vi "Create Pattern Script(OM).vi"(8 "error in (no error)":errorcluster, 10 "BML OM":T1, 11 "BML Pattern Creater in":refnum<class "BML Pattern Creater.lvclass">) -> (0 "error out":errorcluster, 2 "OM string out":string, 3 "BML Pattern Creater out":refnum<class "BML Pattern Creater.lvclass">)   [LabVIEW 2018, in "BML Pattern Creater.lvlib" / "BML Pattern Creater.lvclass"]
uses:
  BML Pattern Creater.lvclass
  Ctls/OM - BML.ctl
  Interfaces/Protocol Interface.lvlibp/Interfaces/Protocol Interface/Pin State.ctl
  Interfaces/Protocol Interface.lvlibp/Interfaces/Protocol Interface/Protocol Interface.lvclass
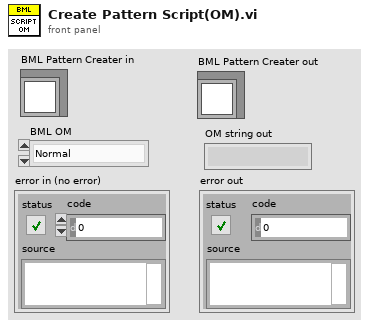
[diagram p1: front panel]
types:
  T1 = typedef "OM - BML.ctl" = enum16{"Normal", "ImmeEffect", "InitSlaveID", "LoadData"}
  T2 = typedef "Protocol Interface.lvlibp/Protocol Interface.lvclass/Pin State.ctl" = enum16{"0", "1", "L", "H", "X", "V", "D", "M"}
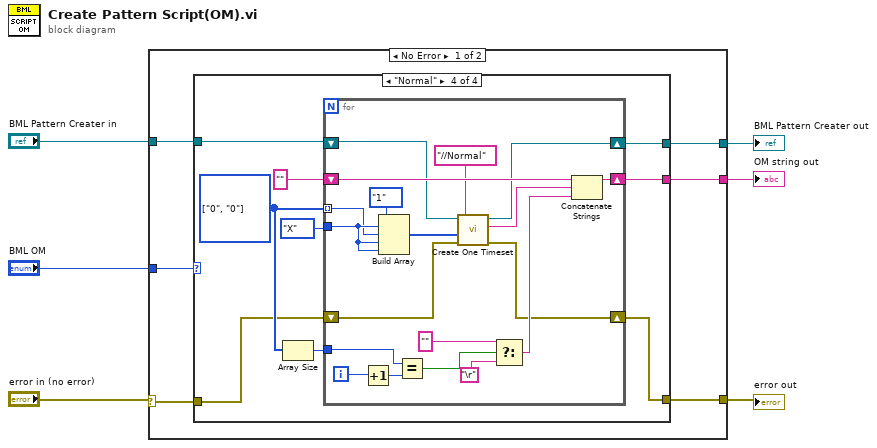
[diagram p0: block diagram]
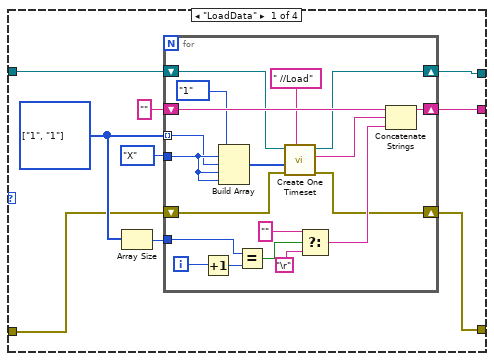
[diagram p2: hidden frame]
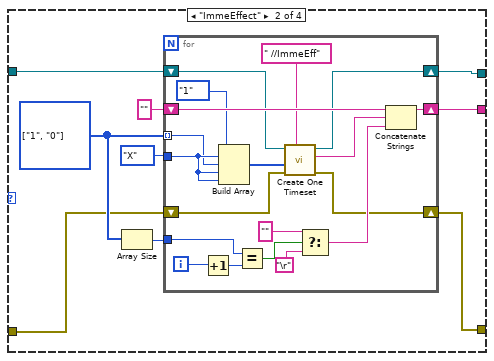
[diagram p3: hidden frame]
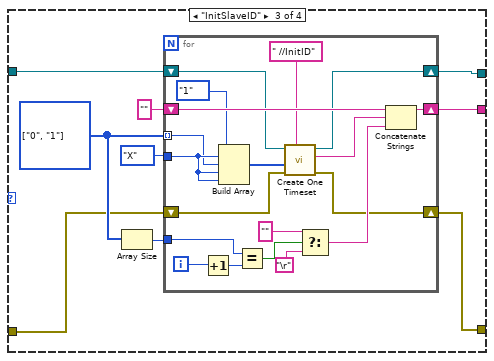
[diagram p4: hidden frame]
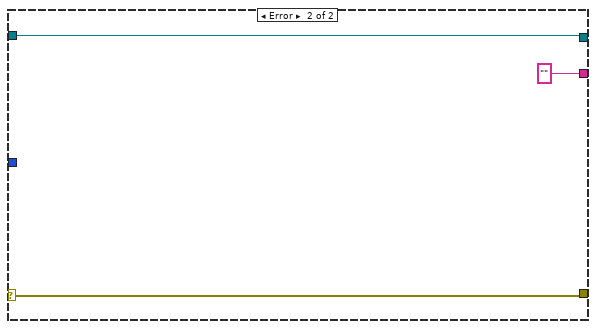
[diagram p5: hidden frame]
diagram:
  n1 = case shown="No Error" "error in (no error)" {
    selector: "error in (no error)" -> [w10 w126]
    tunnel: "BML OM" -> [w12 _]
    tunnel: [w11 "" ("string out")] -> w5
    tunnel: [w9 w126] -> w4
    tunnel: "BML Pattern Creater in" -> [w8 w125]
    tunnel: [w7 w125] -> w1
    frame No Error {
      n2 = case shown="\"Normal\"" w12 {
        tunnel: [w20 w48 w76 w104] -> w11
        tunnel: w10 -> [w16 w44 w72 w100]
        tunnel: [w14 w42 w70 w99] -> w9
        tunnel: w8 -> [w15 w43 w71 w97]
        tunnel: [w13 w41 w69 w98] -> w7
        frame "LoadData" {
          w19 = T2[] [enum."1", enum."1"] items=["0", "1", "L", "H", "X", "V", "D", "M"] ("PinState")
          n3 = Array Size(array=w19) -> (size(s)=w18:i32)
          n4 = for {
            tunnel: w19 -> [w30] mode=indexing
            shift-right: [w39] -> w20
            shift-left: "" ("string out") -> [w40]
            tunnel: w18 -> [w37]
            tunnel: Pin_State."X" ("PinState") -> [w31]
            shift-right: [w24] -> w14
            shift-left: w16 -> [w25]
            shift-right: [w22] -> w13
            shift-left: w15 -> [w23]
            i -> [w38]
            n5 = Increment(x=w38) -> (x+1=w36:i32)
            n6 = Build Array(Pin_State."1" ("PinState"), w31, w30, w31, w31) -> (w26:T2[])
            n7 = Equal?(x=w37, y=w36) -> (x = y?=w35:bool)
            n8 = call-dynamic "Create One Timeset.vi"("Notes"=" //Load", "error in (no error)"=w25, "Pin State"=w26, "BML Pattern Creater in"=w23) -> ("error out"=w24:errorcluster, "string out"=w27:string, "BML Pattern Creater out"=w22:refnum<class "BML Pattern Creater.lvclass">)  [unwired: 5 in]
            n9 = Select(t="", s=w35, f="\r") -> (s? t:f=w32:string)
            n10 = Concatenate Strings(w40, w27, w32) -> (w39:string)
          }
        }
        frame "ImmeEffect" {
          w47 = T2[] [enum."1", enum."0"] items=["0", "1", "L", "H", "X", "V", "D", "M"] ("PinState")
          n11 = Array Size(array=w47) -> (size(s)=w46:i32)
          n12 = for {
            tunnel: w47 -> [w58] mode=indexing
            shift-right: [w67] -> w48
            shift-left: "" ("string out") -> [w68]
            tunnel: w46 -> [w65]
            tunnel: Pin_State."X" ("PinState") -> [w59]
            shift-right: [w52] -> w42
            shift-left: w44 -> [w53]
            shift-right: [w50] -> w41
            shift-left: w43 -> [w51]
            i -> [w66]
            n13 = Increment(x=w66) -> (x+1=w64:i32)
            n14 = Build Array(Pin_State."1" ("PinState"), w59, w58, w59, w59) -> (w54:T2[])
            n15 = Equal?(x=w65, y=w64) -> (x = y?=w63:bool)
            n16 = call-dynamic "Create One Timeset.vi"("Notes"=" //ImmeEff", "error in (no error)"=w53, "Pin State"=w54, "BML Pattern Creater in"=w51) -> ("error out"=w52:errorcluster, "string out"=w55:string, "BML Pattern Creater out"=w50:refnum<class "BML Pattern Creater.lvclass">)  [unwired: 5 in]
            n17 = Select(t="", s=w63, f="\r") -> (s? t:f=w60:string)
            n18 = Concatenate Strings(w68, w55, w60) -> (w67:string)
          }
        }
        frame "InitSlaveID" {
          w75 = T2[] [enum."0", enum."1"] items=["0", "1", "L", "H", "X", "V", "D", "M"] ("PinState")
          n19 = Array Size(array=w75) -> (size(s)=w74:i32)
          n20 = for {
            tunnel: w75 -> [w86] mode=indexing
            shift-right: [w95] -> w76
            shift-left: "" ("string out") -> [w96]
            tunnel: w74 -> [w93]
            tunnel: Pin_State."X" ("PinState") -> [w87]
            shift-right: [w80] -> w70
            shift-left: w72 -> [w81]
            shift-right: [w78] -> w69
            shift-left: w71 -> [w79]
            i -> [w94]
            n21 = Increment(x=w94) -> (x+1=w92:i32)
            n22 = Build Array(Pin_State."1" ("PinState"), w87, w86, w87, w87) -> (w82:T2[])
            n23 = Equal?(x=w93, y=w92) -> (x = y?=w91:bool)
            n24 = call-dynamic "Create One Timeset.vi"("Notes"=" //InitID", "error in (no error)"=w81, "Pin State"=w82, "BML Pattern Creater in"=w79) -> ("error out"=w80:errorcluster, "string out"=w83:string, "BML Pattern Creater out"=w78:refnum<class "BML Pattern Creater.lvclass">)  [unwired: 5 in]
            n25 = Select(t="", s=w91, f="\r") -> (s? t:f=w88:string)
            n26 = Concatenate Strings(w96, w83, w88) -> (w95:string)
          }
        }
        frame "Normal" {
          w103 = T2[] [enum."0", enum."0"] items=["0", "1", "L", "H", "X", "V", "D", "M"] ("PinState")
          n27 = Array Size(array=w103) -> (size(s)=w102:i32)
          n28 = for {
            tunnel: w103 -> [w114] mode=indexing
            shift-right: [w123] -> w104
            shift-left: "" ("string out") -> [w124]
            tunnel: w102 -> [w121]
            tunnel: Pin_State."X" ("PinState") -> [w115]
            shift-right: [w108] -> w99
            shift-left: w100 -> [w109]
            shift-right: [w107] -> w98
            shift-left: w97 -> [w106]
            i -> [w122]
            n29 = Increment(x=w122) -> (x+1=w120:i32)
            n30 = Build Array(Pin_State."1" ("PinState"), w115, w114, w115, w115) -> (w110:T2[])
            n31 = Equal?(x=w121, y=w120) -> (x = y?=w119:bool)
            n32 = call-dynamic "Create One Timeset.vi"("Notes"="//Normal", "error in (no error)"=w109, "Pin State"=w110, "BML Pattern Creater in"=w106) -> ("error out"=w108:errorcluster, "string out"=w111:string, "BML Pattern Creater out"=w107:refnum<class "BML Pattern Creater.lvclass">)  [unwired: 5 in]
            n33 = Select(t="", s=w119, f="\r") -> (s? t:f=w116:string)
            n34 = Concatenate Strings(w124, w111, w116) -> (w123:string)
          }
        }
      }
    }
    frame Error {
    }
  }
  "error out" <- w4
  "OM string out" <- w5
  "BML Pattern Creater out" <- w1
